vi "fsffsfs.vi"() -> ()   [LabVIEW 2015]
uses:
  <vilib>/NXT/Block Support/NXT_InputPort.ctl
  <vilib>/NXT/Subs/MotorOutput.ctl
  <vilib>/NXT/Dual Mode Library/Sensors/Sonar_cm.vi
  <vilib>/NXT/Dual Mode Library/Motors/MotorOn.vi
  <vilib>/NXT/Dual Mode Library/Sensors/Light_On.vi
  <vilib>/NXT/Dual Mode Library/Motors/MotorReverse.vi
  <vilib>/NXT/Dual Mode Library/Waits/Wait_Num.vi
panel:
  in  "沥瘤":bool
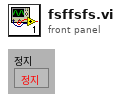
[diagram p1: front panel]
types:
  T1 = typedef "MotorOutput.ctl" = u8
  T2 = typedef "NXT_InputPort.ctl" = u32
  T3 = typedef "LVHSConnector.ctl" = refnum<class "BrickReference.lvclass">
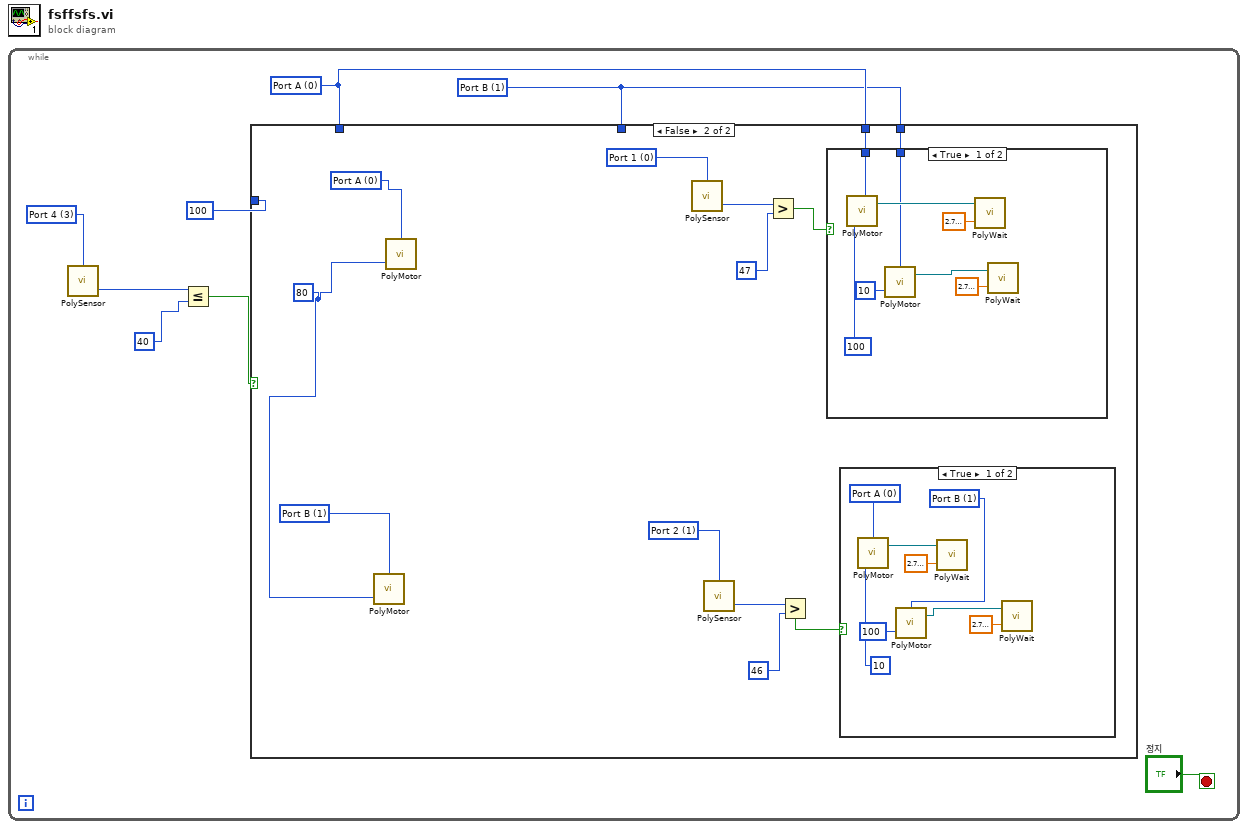
[diagram p0: block diagram]
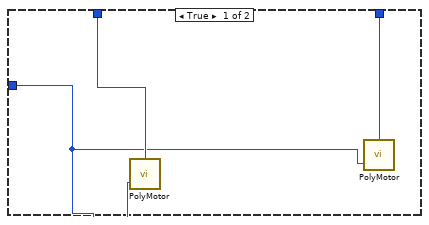
[diagram p2: hidden frame]
diagram:
  n1 = while {
    stop <- "沥瘤" stop-if-true
    w1 = T1 1 items=["Port A", "Port B", "Port C", "All Ports"] ("Output Port (All Ports)")
    w2 = T1 0 items=["Port A", "Port B", "Port C", "All Ports"] ("Output Port (All Ports)")
    w5 = T2 3 items=["Port 1", "Port 2", "Port 3", "Port 4"] ("Input Port")
    n2 = call-poly <vilib>:"PolySensor.vi"("Port (Port 4)"=w5) -> ("Distance (cm)"=w3:i16)  [unwired: 2 in, 1 out]
    n3 = Less Or Equal?(x=w3, y=40) -> (x <= y?=w6:bool)
    n4 = case shown="False" w6 {
      tunnel: w2 -> [w11 _]
      tunnel: 100 ("Power (75)") -> [w9 _]
      tunnel: w1 -> [w10 _]
      tunnel: w2 -> [_ w15]
      tunnel: w1 -> [_ w14]
      frame True {
        n5 = call-poly <vilib>:"PolyMotor.vi"("Power (75)"=w9, "Output Port (All Ports)"=w11) -> ()  [unwired: 2 in, 1 out]
        n6 = call-poly <vilib>:"PolyMotor.vi"("Power (75)"=w9, "Output Port (All Ports)"=w10) -> ()  [unwired: 2 in, 1 out]
      }
      frame False {
        w13 = T1 1 items=["Port A", "Port B", "Port C", "All Ports"] ("Output Port (All Ports)")
        w17 = T2 1 items=["Port 1", "Port 2", "Port 3", "Port 4"] ("Input Port")
        w16 = T2 0 items=["Port 1", "Port 2", "Port 3", "Port 4"] ("Input Port")
        w12 = 80 ("Power (75)")
        w24 = T1 0 items=["Port A", "Port B", "Port C", "All Ports"] ("Output Port (All Ports)")
        n7 = call-poly <vilib>:"PolyMotor.vi"("Power (75)"=w12, "Output Port (All Ports)"=w13) -> ()  [unwired: 2 in, 1 out]
        n8 = call-poly <vilib>:"PolyMotor.vi"("Power (75)"=w12, "Output Port (All Ports)"=w24) -> ()  [unwired: 2 in, 1 out]
        n9 = call-poly <vilib>:"PolySensor.vi"("Port (Port 3)"=w16) -> ("Scaled Value"=w20:i16)  [unwired: 2 in, 1 out]
        n10 = call-poly <vilib>:"PolySensor.vi"("Port (Port 3)"=w17) -> ("Scaled Value"=w23:i16)  [unwired: 2 in, 1 out]
        n11 = Greater?(x=w20, y=47) -> (0:w18:bool)
        n12 = Greater?(x=w23, y=46) -> (0:w21:bool)
        n13 = case shown="True" w18 {
          tunnel: w15 -> [w30 _]
          tunnel: w14 -> [w26 _]
          frame True {
            n14 = call-poly <vilib>:"PolyMotor.vi"("Power (75)"=100, "Output Port (All Ports)"=w30) -> ("NXT/EV3"=w32:T3)  [unwired: 2 in]
            n15 = call-poly <vilib>:"PolyMotor.vi"("Power (75)"=10, "Output Port (All Ports)"=w26) -> ("NXT/EV3"=w28:T3)  [unwired: 2 in]
            n16 = call-poly <vilib>:"PolyWait.vi"("Time (1 sec)"=sgl 2.7 ("Time (sec)"), "NXT/EV3"=w32) -> ()  [unwired: 2 in, 1 out]
            n17 = call-poly <vilib>:"PolyWait.vi"("Time (1 sec)"=sgl 2.7 ("Time (sec)"), "NXT/EV3"=w28) -> ()  [unwired: 2 in, 1 out]
          }
          frame False {
          }
        }
        n18 = case shown="True" w21 {
          frame True {
            w35 = T1 1 items=["Port A", "Port B", "Port C", "All Ports"] ("Output Port (All Ports)")
            w38 = T1 0 items=["Port A", "Port B", "Port C", "All Ports"] ("Output Port (All Ports)")
            n19 = call-poly <vilib>:"PolyMotor.vi"("Power (75)"=10, "Output Port (All Ports)"=w38) -> ("NXT/EV3"=w40:T3)  [unwired: 2 in]
            n20 = call-poly <vilib>:"PolyMotor.vi"("Power (75)"=100, "Output Port (All Ports)"=w35) -> ("NXT/EV3"=w36:T3)  [unwired: 2 in]
            n21 = call-poly <vilib>:"PolyWait.vi"("Time (1 sec)"=sgl 2.7 ("Time (sec)"), "NXT/EV3"=w40) -> ()  [unwired: 2 in, 1 out]
            n22 = call-poly <vilib>:"PolyWait.vi"("Time (1 sec)"=sgl 2.7 ("Time (sec)"), "NXT/EV3"=w36) -> ()  [unwired: 2 in, 1 out]
          }
          frame False {
          }
        }
      }
    }
  }
